vi "Gen CRC-16.vi"(8 "error in (no error)":errorcluster caption="error in（no error）", 11 "Data In":u8[](array[numeric]) format="%.0x") -> (0 "error out":errorcluster, 1 "CRC-16-H":u8 format="%.0x", 2 "CRC-16-L":u8 format="%.0x", 3 "CRC-16-Result":u16 format="%.0x")   [LabVIEW 2014, in "ALPHA5 RS485.lvlib"]
uses:
  ALPHA5 RS485.lvlib
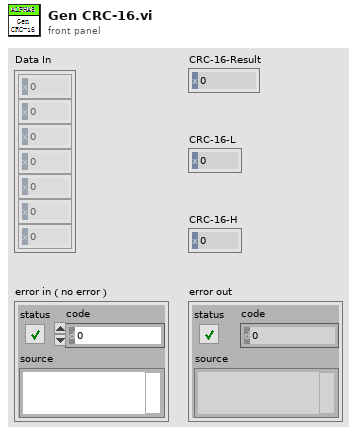
[diagram p1: front panel]
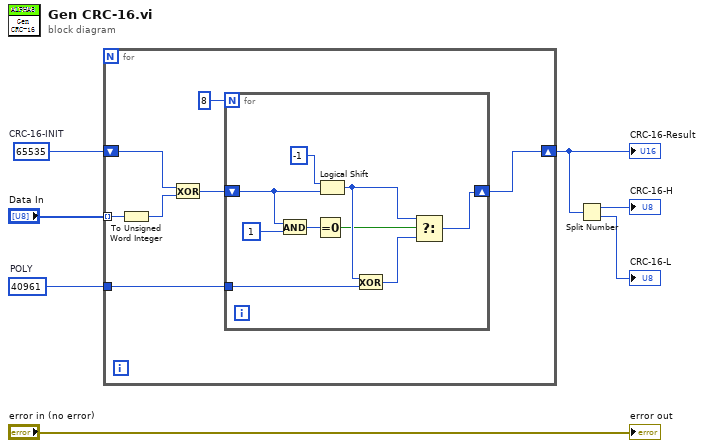
[diagram p0: block diagram]
diagram:
  w5 = u16 40961  # POLY
  w6 = u16 65535  # CRC-16-INIT
  n1 = for {
    tunnel: "Data In" -> [w13] mode=indexing
    tunnel: w5 -> [w9]
    shift-right: [w8] -> w3
    shift-left: w6 -> [w14]
    n2 = To Unsigned Word Integer(number=w13) -> (unsigned 16bit integer=w12:u16)
    n3 = Exclusive Or(1:w12, 2:w14) -> (0:w10:u16)
    n4 = for {
      N: 8 -> [_]
      tunnel: w9 -> [w22]
      shift-right: [w20] -> w8
      shift-left: w10 -> [w16]
      n5 = And(x=w16, y=u16 1) -> (x .and. y?=w18:u16)
      n6 = Equal To 0?(x=w18) -> (x = 0?=w15:bool)
      n7 = Logical Shift(y=i16 -1, x=w16) -> (x << y=w19:u16)
      n8 = Exclusive Or(1:w22, 2:w19) -> (0:w21:u16)
      n9 = Select(t=w19, s=w15, f=w21) -> (s? t:f=w20:u16)
    }
  }
  "CRC-16-Result" <- w3
  n10 = Split Number(x=w3) -> (hi(x)=→"CRC-16-H":u8, lo(x)=→"CRC-16-L":u8)
  "error out" <- "error in (no error)"
